vi "Untitled 15.vi"() -> ()   [LabVIEW 2019]
uses:
  Generated_client/RPC Messages/Greeter_req.ctl
  Generated_client/RPC Messages/Greeter_req_req_oneof/Greeter_req_req_oneof.lvclass
  Generated_client/RPC Messages/Greeter_res_res_oneof/Greeter_res_res_oneof.lvclass
  Generated_client/RPC Messages/Greeter_req_req_oneof/Greeter_req_req_oneof.lvclass/Greeter_req_req_oneof.ctl
  Generated_client/RPC Messages/Greeter_res_res_oneof/Greeter_res_res_oneof.lvclass/Greeter_res_res_oneof.ctl
  Generated_client/Generated_client.lvlib
panel:
  out "OneOfTemplate out":refnum<class "Greeter_res_res_oneof.lvclass">
  out "Get_Val":bool
  out "error out 2":errorcluster
  in  "error in (no error)":errorcluster
  in  "Set_Val":bool
  out "res_latitude":i32
  out "error out":errorcluster
  in  "Request Data":T1
  in  "address":string
  in  "error in":errorcluster
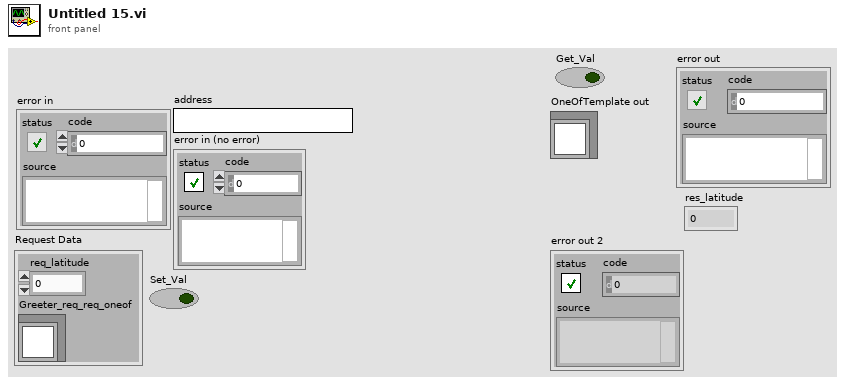
[diagram p1: front panel]
types:
  T1 = typedef "Generated_client.lvlib/Greeter_req.ctl" = cluster{"req_latitude":i32, "Greeter_req_req_oneof":refnum<class "Greeter_req_req_oneof.lvclass">}
  T2 = typedef "grpc-lvsupport-release.lvlib/grpcId.ctl" = u64
  T3 = typedef "Generated_client.lvlib/Greeter_res.ctl" = cluster{"res_latitude":i32, "Greeter_res_res_oneof":refnum<class "Greeter_res_res_oneof.lvclass">}
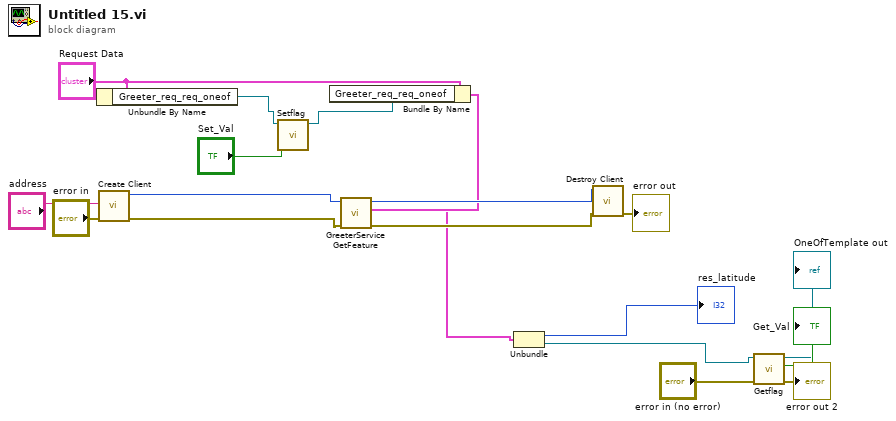
[diagram p0: block diagram]
diagram:
  n1 = Unbundle By Name("Request Data") -> ("Greeter_req_req_oneof"=w8:refnum<class "Greeter_req_req_oneof.lvclass">)
  n2 = call "Create Client.vi"("error in"="error in", "address"="address") -> ("error out"=w17:errorcluster, "gRPC ID Out"=w19:T2)  [unwired: 8 in]
  n3 = call "Setflag.vi"("Set_Val"="Set_Val", "OneOfTemplate in"=w8) -> ("OneOfTemplate out"=w7:refnum<class "Greeter_req_req_oneof.lvclass">)  [unwired: 8 in, 1 out]
  n4 = Bundle By Name(cluster="Request Data", "Greeter_req_req_oneof"=w7) -> (w11:T1)
  n5 = call "GreeterService GetFeature.vi"("error in"=w17, "Request Data"=w11, "gRPC ID"=w19) -> ("error out"=w16:errorcluster, "Response Data"=w10:T3, "gRPC ID out"=w18:T2)  [unwired: 6 in]
  n6 = Unbundle(w10) -> ("res_latitude"=→"res_latitude":i32, "Greeter_res_res_oneof"=w5:refnum<class "Greeter_res_res_oneof.lvclass">)
  n7 = call "Destroy Client.vi"("error in"=w16, "gRPC ID"=w18) -> ("error out"=→"error out":errorcluster)  [unwired: 9 in]
  n8 = call "Getflag.vi"("error in (no error)"="error in (no error)", "OneOfTemplate in"=w5) -> ("error out"=→"error out 2":errorcluster, "Get_Val"=→"Get_Val":bool, "OneOfTemplate out"=→"OneOfTemplate out":refnum<class "Greeter_res_res_oneof.lvclass">)  [unwired: 7 in]
